vi "SQL_CycleTime_RegisterMachine.vi"(8 "MachineName":string, 9 "LineName":string, 10 "TableName":string, 11 "ConnectionDSN":string) -> ()   [LabVIEW 2017]
uses:
  <vilib>/addons/database/Connection.llb/DB Tools Open Connec (String).vi
  <vilib>/addons/database/Connection.llb/Conn Execute.vi
  <vilib>/addons/database/NI_Database_API.lvlib
panel:
  in  "Date":string
  in  "CycleTime":string
  # "This VI updates the cycle time live in the database"
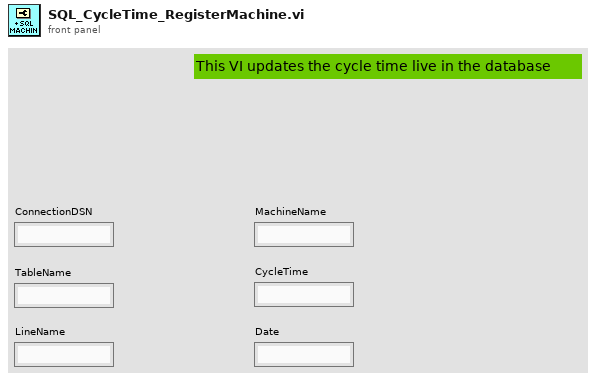
[diagram p1: front panel]
types:
  T1 = typedef "NI_Database_API.lvlib/Conn ObjectReference.ctl" = refnum<k1>
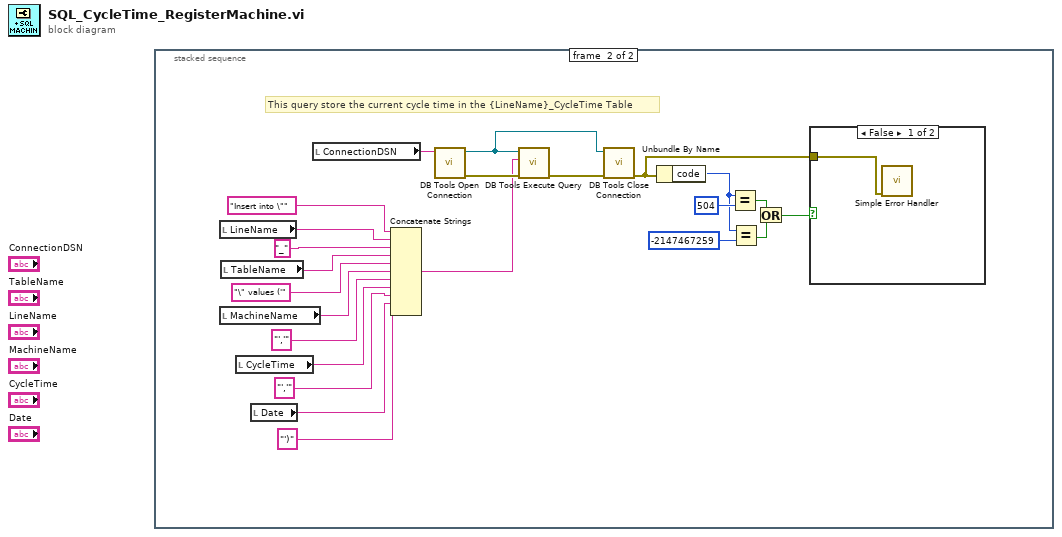
[diagram p0: block diagram]
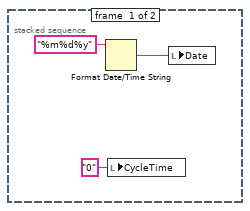
[diagram p2: hidden frame]
diagram:
  n1 = stacked-sequence {
    frame #0 {
      n2 = Format Date/Time String(time format string (%c)="%m%d%y") -> (date/time string=w3:string)  [unwired: 2 in]
      n3 = local write "CycleTime"("0" ("CycleTime")) -> ()
      n4 = local write "Date"(w3) -> ()
    }
    frame #1 {
      # "This query store the current cycle time in the {LineName}_CycleTime Table"
      n5 = local read "LineName"() -> (w21:string)
      n6 = local read "MachineName"() -> (w17:string)
      n7 = local read "TableName"() -> (w19:string)
      n8 = local read "CycleTime"() -> (w15:string)
      n9 = local read "Date"() -> (w13:string)
      n10 = local read "ConnectionDSN"() -> (w26:string)
      n11 = Concatenate Strings("Insert into \"", w21, "_", w19, "\" values ('", w17, "','", w15, "','", w13, "')") -> (w11:string)
      n12 = call-poly <vilib>:"DB Tools Open Connection.vi"("connection information"=w26) -> ("error out"=w25:errorcluster, "connection reference"=w23:T1)  [unwired: 7 in]
      n13 = call-poly <vilib>:"DB Tools Execute Query.vi"("error in (no error)"=w25, "SQL query"=w11, "connection reference"=w23) -> ("error out"=w24:errorcluster)  [unwired: 5 in, 1 out]
      n14 = call <vilib>:"DB Tools Close Connection.vi"("error in (no error)"=w24, "connection reference"=w23) -> ("error out"=w9:errorcluster)  [unwired: 5 in]
      n15 = Unbundle By Name(w9) -> ("code"=w8:i32)
      n16 = Equal?(x=w8, y=504) -> (x = y?=w6:bool)
      n17 = Equal?(x=w8, y=-2147467259) -> (x = y?=w5:bool)
      n18 = Or(x=w6, y=w5) -> (x .or. y?=w4:bool)
      n19 = case shown="False" w4 {
        tunnel: w9 -> [w27 _]
        frame False {
          n20 = call <vilib>:"Simple Error Handler.vi"("error in (no error)"=w27) -> ()  [unwired: 4 in, 5 out]
        }
        frame True {
        }
      }
    }
  }
